vi "CSMOMgr-Update CSMO.vi"(8 "error in (no error)":errorcluster, 10 "CSMO":T1={"Requested Name"="", "Module Name"="", "Mode"=enum."Stand Alone", "Queue"=refnum, "CSM-Data"=refnum, "User Event"=refnum, "Status Change Event"=refnum, "Allowed Messages"=[], "Mode-Data"=refnum, "Group Name"="", "Exit Event"=refnum}, 11 "CSMOMgr in":T3) -> (0 "error out":errorcluster, 2 "CSMO(dup)":T1={"Requested Name"="", "Module Name"="", "Mode"=enum."Stand Alone", "Queue"=refnum, "CSM-Data"=refnum, "User Event"=refnum, "Status Change Event"=refnum, "Allowed Messages"=[], "Mode-Data"=refnum, "Group Name"="", "Exit Event"=refnum}, 3 "CSMOMgr out":T3)   [LabVIEW 2020, in "Communicable State Machine.lvlib"]
uses:
  Communicable State Machine.lvlib
  _CSMObj.ctl
  Priority Queue.lvclass
  _CSM_MODE.ctl
  _CSMObj-Data.ctl
  _CSM Status Change Event Data.ctl
  _CSMObj-ModeData.ctl
  Def-CSMOMgr.ctl
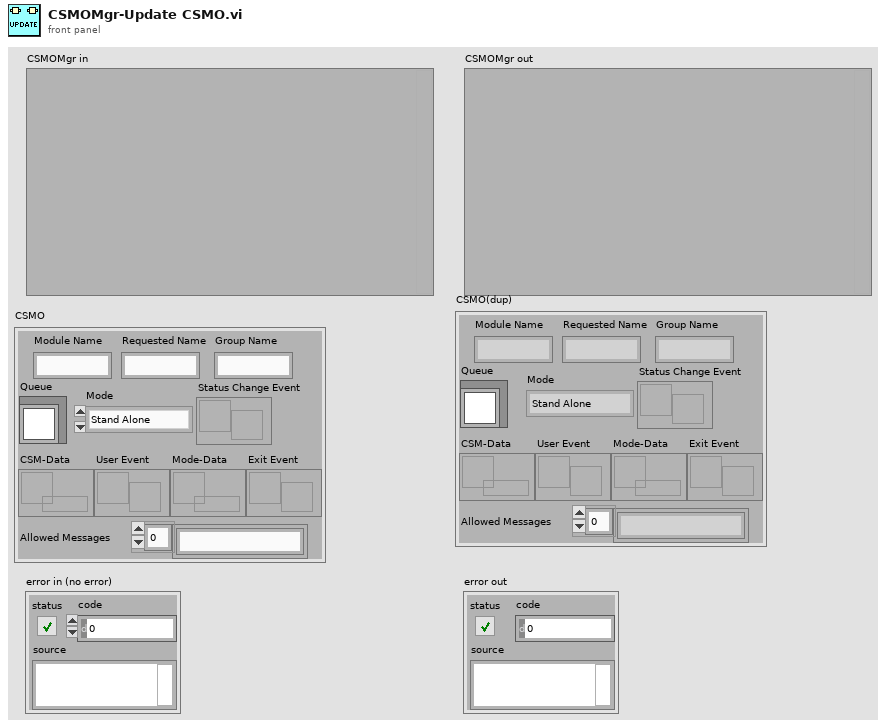
[diagram p1: front panel]
types:
  T1 = typedef "Communicable State Machine.lvlib/_CSMObj.ctl" = cluster{"Requested Name":string, "Module Name":string, "Mode":T2, "Queue":refnum<class "Priority Queue.lvclass">, "CSM-Data":refnum<data-value>, "User Event":refnum<user-event>, "Status Change Event":refnum<user-event>, "Allowed Messages":string[], "Mode-Data":refnum<data-value>, "Group Name":string, "Exit Event":refnum<user-event>}
  T2 = typedef "Communicable State Machine.lvlib/_CSM_MODE.ctl" = enum16{"Not Exist", "Stand Alone", "CSM", "Worker Agent", "Worker", "Chain", "Chain Node"}
  T3 = typedef "Communicable State Machine.lvlib/Def-CSMOMgr.ctl" = variant
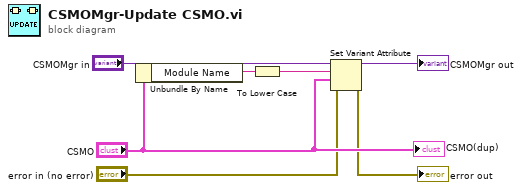
[diagram p0: block diagram]
diagram:
  n1 = Unbundle By Name("CSMO") -> ("Module Name"=w6:string)
  n2 = To Lower Case(string=w6) -> (all lower case string=w1:string)
  n3 = Set Variant Attribute(Variant="CSMOMgr in", name=w1, value="CSMO", error in="error in (no error)") -> (Variant out=→"CSMOMgr out":T3, error out=→"error out":errorcluster)  [unwired: 1 out]
  "CSMO(dup)" <- "CSMO"
